vi "Execute Rewind Button.vi"(0 "reference in":refnum<class "Client.lvclass">, 11 "Error In":errorcluster) -> (4 "reference out":refnum<class "Client.lvclass">, 15 "Error Out":errorcluster)   [LabVIEW 2024, in "Client.lvclass"]
uses:
  Client.lvclass
  Invoker/RemoteControl_class/RemoteControl.lvclass
panel:
  # "Connector Pane"
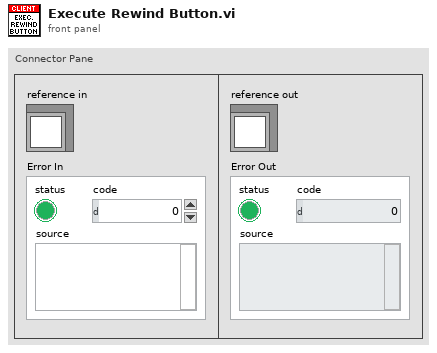
[diagram p1: front panel]
types:
  T1 = typedef "Client.lvclass/ObjectAttributes.ctl" = cluster{"RemoteControlRef":refnum<class "RemoteControl.lvclass">, "MediaPlayerRef":refnum<class "MediaPlayer.lvclass">, "Commands":cluster{"Play Music Command":refnum<class "IPlayerCommand.lvclass">, "Pause Music Command":refnum<class "IPlayerCommand.lvclass">, "Stop Music Command":refnum<class "IPlayerCommand.lvclass">, "Skip Music Command":refnum<class "IPlayerCommand.lvclass">, "Get Current Info Command":refnum<class "IPlayerCommand.lvclass">, "Rewind Music Command":refnum<class "IPlayerCommand.lvclass">}}
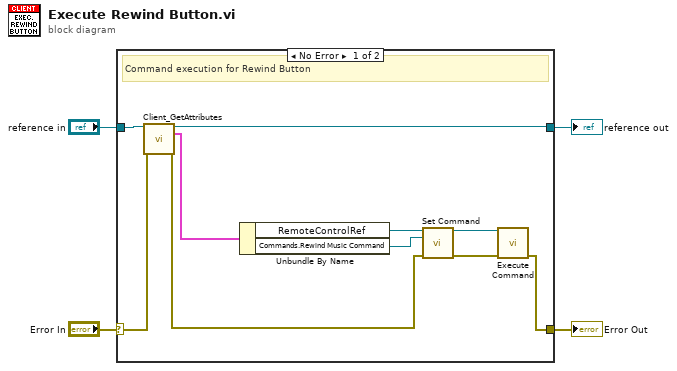
[diagram p0: block diagram]
diagram:
  n1 = case shown="No Error" "Error In" {
    selector: "Error In" -> [w14 w16]
    tunnel: [w9 w16] -> w3
    tunnel: [w11 w15] -> w1
    tunnel: "reference in" -> [w12 w15]
    frame No Error {
      # "Command execution for Rewind Button"
      n2 = call "Client_GetAttributes.vi"("reference in"=w12, "Error In"=w14) -> ("reference out"=w11:refnum<class "Client.lvclass">, "Data"=w13:T1, "Error Out"=w10:errorcluster)  [unwired: 10 in, 1 out]
      n3 = Unbundle By Name(w13) -> ("RemoteControlRef"=w7:refnum<class "RemoteControl.lvclass">, "Commands.Rewind Music Command"=w5:refnum<class "IPlayerCommand.lvclass">)
      n4 = call-dynamic "Set Command.vi"("reference in"=w7, "Command"=w5, "Error In"=w10) -> ("reference out"=w6:refnum<class "RemoteControl.lvclass">, "Error Out"=w8:errorcluster)  [unwired: 11 in]
      n5 = call-dynamic "Execute Command.vi"("reference in"=w6, "Error In"=w8) -> ("Error Out"=w9:errorcluster)  [unwired: 12 in, 1 out]
    }
    frame Error {
    }
  }
  "Error Out" <- w3
  "reference out" <- w1
